vi "SI8.vi"(4 "error in":T13, 7 "Command":T14) -> (0 "error out":T13, 3 "Response":T11)   [LabVIEW 2018]
uses:
  MOKO_LabViewLibrary/MokoLowLevel/MokoLowLovelControl/MLLC_Command.ctl
  MOKO_LabViewLibrary/MokoLowLevel/MokoLowLovelControl/MLLC_Error.ctl
  MOKO_LabViewLibrary/MokoLowLevel/MokoLowLovelControl/MLLC_Mode.ctl
  MOKO_LabViewLibrary/MokoLowLevel/MokoLowLovelControl/MLLC_Response.ctl
  MOKO_LabViewLibrary/MokoLowLevel/MokoLowLovelControl/MLLC_DriverName.ctl
  MOKO_LabViewLibrary/MokoLowLevel/MokoLowLovelControl/MLLC_ResponseInit.ctl
  MOKO_LabViewLibrary/MokoLowLevel/MokoLowLovelControl/MLLC_Request.ctl
  MOKO_LabViewLibrary/MokoLowLevel/MokoLowLovelControl/MLLC_ErrorCode.ctl
  MOKO_LabViewLibrary/MokoLowLevel/MokoLowLovelControl/MLLC_ConnectCluster.ctl
  MOKO_LabViewLibrary/MokoLowLevel/MokoLowLovelControl/MLLC_InterfaceType.ctl
  MOKO_LabViewLibrary/MokoLowLevel/MokoLowLovelControl/MLLC_OpenedSession.ctl
  MOKO_LabViewLibrary/MokoLowLevel/MokoLowLovelControl/MLLC_InterfaceSettings.ctl
  MOKO_LabViewLibrary/MokoLowLevel/MokoLowLovelControl/MLLC_InterfaceKind.ctl
  MOKO_LabViewLibrary/MokoLowLevel/MokoLowLovelControl/MLLC_Rs232Settings.ctl
panel:
  in  "Settings":T6={"Permanent data"={"Connect"={"InterfaceType"=enum."VISA", "OpenedSession"="COM4", "InterfaceSettings"={"Interface"=enum."RS232", "EOS 4 read"=enum."Default (=EOS 4 write)", "EOS 4 write"=enum."CR (\\r)", "TMO, ms"=2000, "Sett"=variant(cluster{"Baud Rate":u32, "Data Bits":u16, "Parity":u16, "Stop Bits":u16, "Flow Control":u16, "Eho":bool} {"Baud Rate"=75, "Data Bits"=0, "Parity"=0, "Stop Bits"=0, "Flow Control"=0, "Eho"=FALSE})}}}, "Saved Data"=variant}
  in  "Error Code":T7=5420
  in  "Request":T8="?MOD"
  in  "ResponseInit":T9="XP2I"
  in  "Driver Name":T10="Crystal XP2"
  in  "Mode":T12=enum."Check"
  # "SI8"
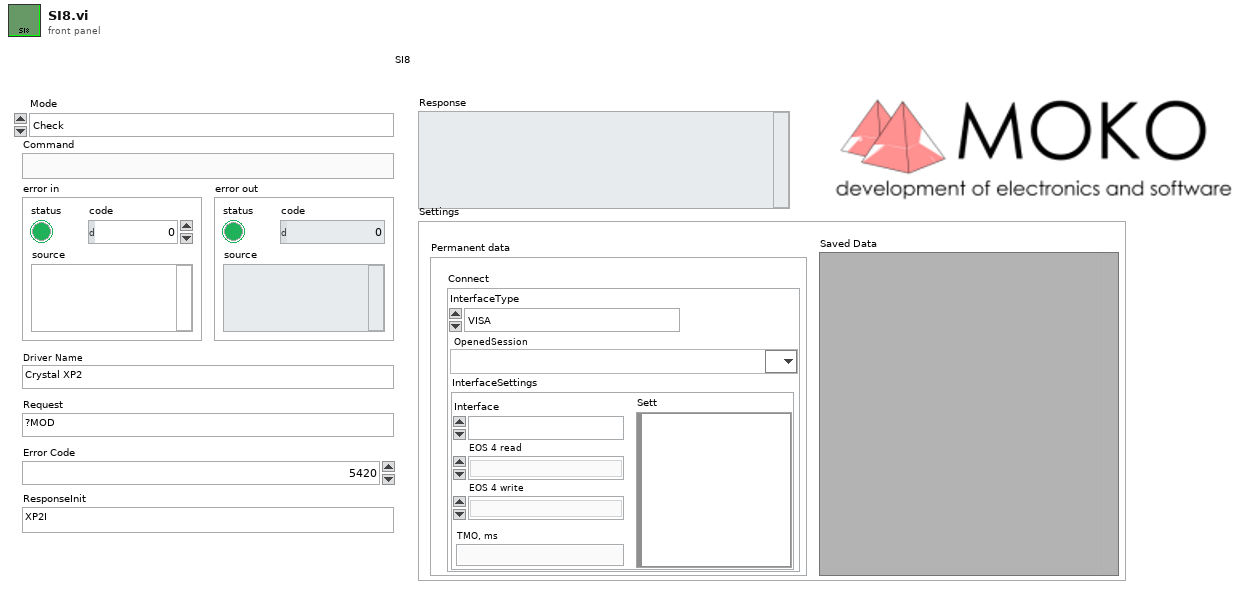
[diagram p1: front panel]
types:
  T1 = typedef "MLLC_ConnectCluster.ctl" = cluster{"InterfaceType":T2, "OpenedSession":T3, "InterfaceSettings":T4}
  T2 = typedef "MLLC_InterfaceType.ctl" = enum16{"VISA", "Prologix USB-GPIB"}
  T3 = typedef "MLLC_OpenedSession.ctl" = refnum<visa-resource-name>
  T4 = typedef "MLLC_InterfaceSettings.ctl" = cluster{"Interface":T5, "EOS 4 read":enum16{"Default (=EOS 4 write)", "CR (\\r)", "LF (\\n)", "None"}, "EOS 4 write":enum16{"CR+LF (\\r\\n)", "CR (\\r)", "LF (\\n)", "None"}, "TMO, ms":i32, "Sett":variant}
  T5 = typedef "MLLC_InterfaceKind.ctl" = enum16{"RS232", "GPIB", "USB", "Ethernet", "another"}
  T6 = cluster{"Permanent data":cluster{"Connect":T1}, "Saved Data":variant}
  T7 = typedef "MLLC_ErrorCode.ctl" = u32
  T8 = typedef "MLLC_Request.ctl" = string
  T9 = typedef "MLLC_ResponseInit.ctl" = string
  T10 = typedef "MLLC_DriverName.ctl" = string
  T11 = typedef "MLLC_Response.ctl" = string
  T12 = typedef "MLLC_Mode.ctl" = enum16{"get", "set", "close", "Init", "Check"}
  T13 = typedef "MLLC_Error.ctl" = errorcluster
  T14 = typedef "MLLC_Command.ctl" = string
  T15 = typedef "MLLC_Rs232Settings.ctl" = cluster{"Baud Rate":u32, "Data Bits":u16, "Parity":u16, "Stop Bits":u16, "Flow Control":u16, "Eho":bool, "Address":dbl}
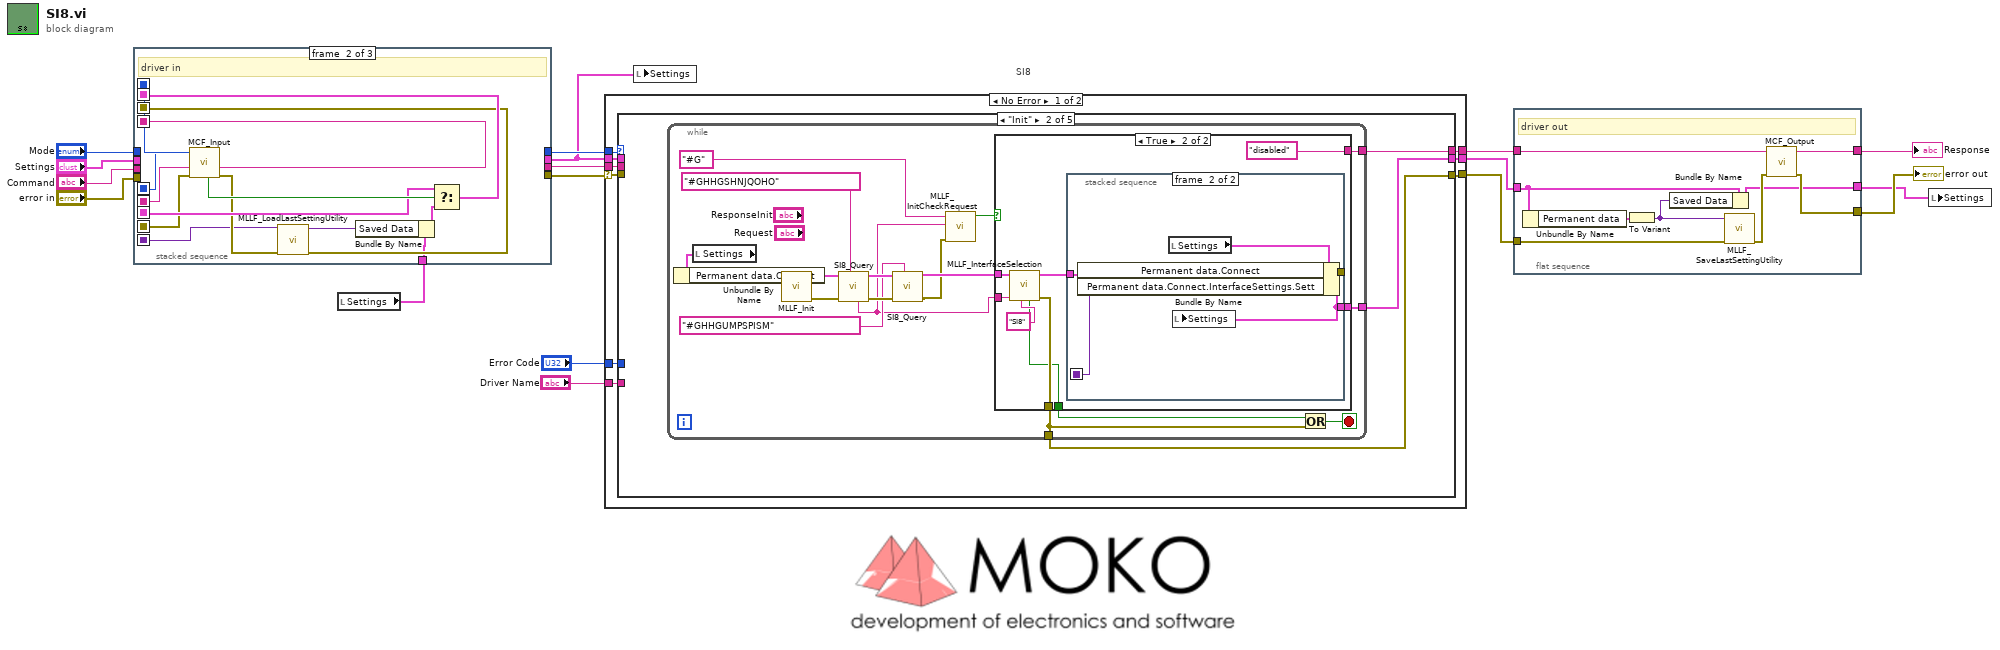
[diagram p0: block diagram]
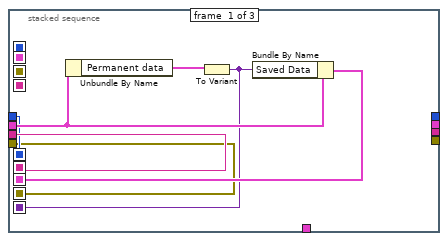
[diagram p2: hidden frame]
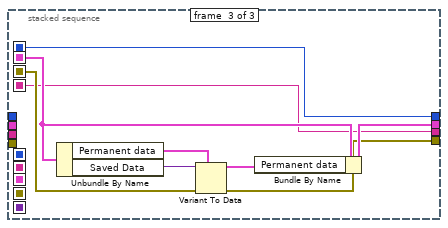
[diagram p3: hidden frame]
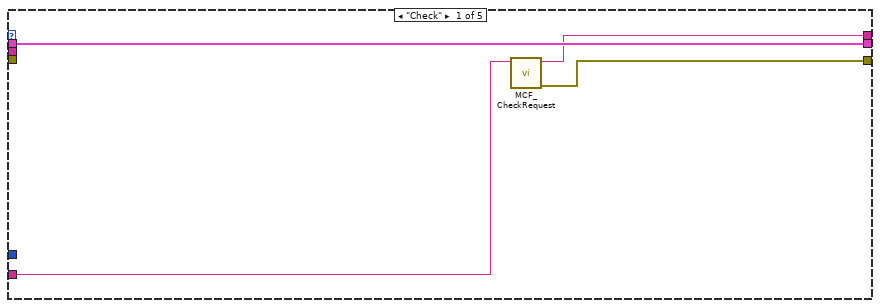
[diagram p4: hidden frame]
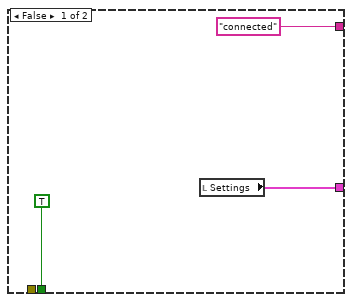
[diagram p5: hidden frame]
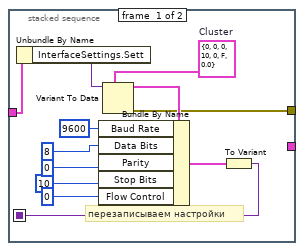
[diagram p6: hidden frame]
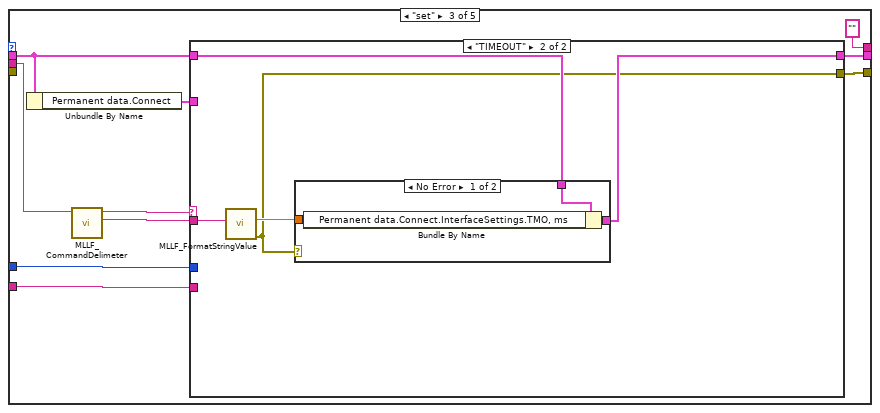
[diagram p7: hidden frame]
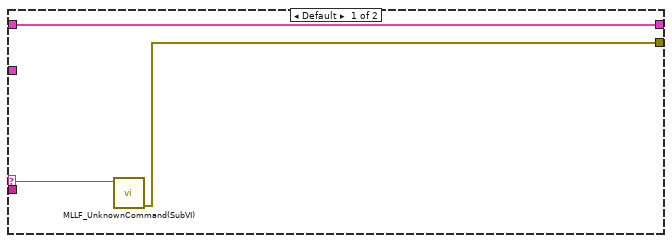
[diagram p8: hidden frame]
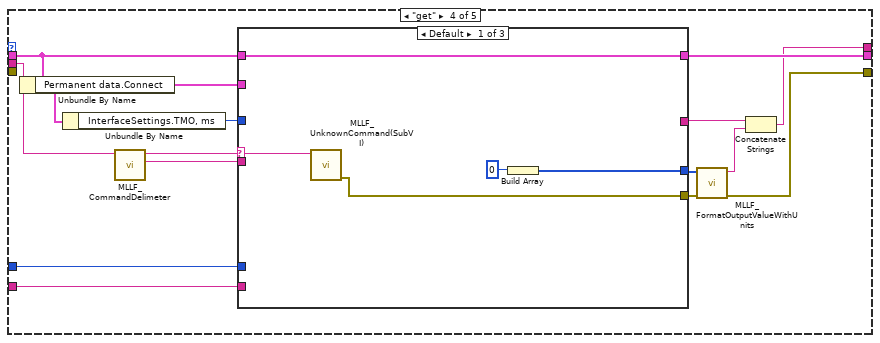
[diagram p10: hidden frame]
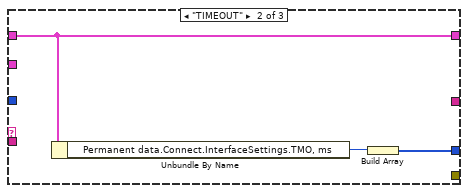
[diagram p11: hidden frame]
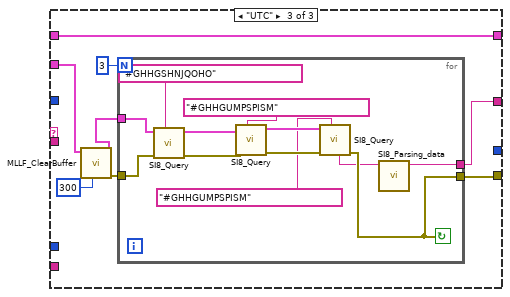
[diagram p12: hidden frame]
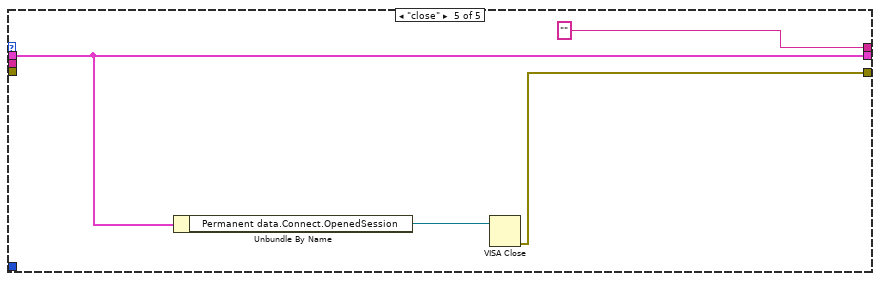
[diagram p13: hidden frame]
diagram:
  # "SI8"
  n1 = local read "Settings"() -> (w7:T6)
  n2 = stacked-sequence {
    seq-local: [w20 _ _] -> [_ w36 _]
    seq-local: [w19 _ _] -> [_ w37 _]
    seq-local: [w22 _ _] -> [_ w32 _]
    seq-local: [w18 _ _] -> [_ w31 _]
    seq-local: [w21 _ _] -> [_ w27 _]
    seq-local: [_ w28 _] -> [_ _ w44]
    seq-local: [_ w38 _] -> [_ _ w41]
    seq-local: [_ w35 _] -> [_ _ w40]
    seq-local: [_ w34 _] -> [_ _ w45]
    tunnel: "Command" -> [w20 _ _]
    tunnel: "Mode" -> [w19 _ _]
    tunnel: "error in" -> [w18 _ _]
    tunnel: "Settings" -> [w23 _ _]
    tunnel: w7 -> [_ w26 _]
    tunnel: [_ _ w40] -> w9
    tunnel: [_ _ w43] -> w10
    tunnel: [_ _ w42] -> w8
    tunnel: [_ _ w41] -> w11
    frame #0 {
      n3 = Unbundle By Name(w23) -> ("Permanent data"=w24:cluster{"Connect":T1})
      n4 = To Variant(anything=w24) -> (Variant=w21:variant)
      n5 = Bundle By Name(cluster=w23, "Saved Data"=w21) -> (w22:T6)
    }
    frame #1 {
      # "driver in"
      n6 = call "MCF_Input.vi"("Error In"=w31, "Command in"=w36, "Mode in"=w37) -> ("Error Out"=w30:errorcluster, "Command out"=w35:string, "Mode out"=w38:T12, "Boolean"=w33:bool)  [unwired: 5 in]
      n7 = call "MLLF_LoadLastSettingUtility.vi"("Error In"=w30, "Save data in"=w27) -> ("Error Out"=w28:errorcluster, "Save data out"=w25:variant)  [unwired: 8 in]
      n8 = Bundle By Name(cluster=w26, "Saved Data"=w25) -> (w29:T6)
      n9 = Select(t=w32, s=w33, f=w29) -> (s? t:f=w34:T6)
    }
    frame #2 {
      n10 = Unbundle By Name(w45) -> ("Permanent data"=w46:cluster{"Connect":T1}, "Saved Data"=w39:variant)
      n11 = Variant To Data(error in=w44, type=w46, Variant=w39) -> (data=w47:cluster{"Connect":T1}, error out=w42:errorcluster)
      n12 = Bundle By Name(cluster=w45, "Permanent data"=w47) -> (w43:T6)
    }
  }
  n13 = case shown="No Error" w8 {
    selector: w8 -> [w53 w179]
    tunnel: [w48 w179] -> w4
    tunnel: w11 -> [w56 _]
    tunnel: [w55 _] -> w6
    tunnel: w9 -> [w54 _]
    tunnel: w10 -> [w50 w178]
    tunnel: "Error Code" -> [w52 _]
    tunnel: "Driver Name" -> [w51 _]
    tunnel: [w49 w178] -> w5
    frame No Error {
      n14 = case shown="\"Init\"" w56 {
        tunnel: [w58 w63 "" ("Output String") w132 "" ("Output String")] -> w55
        tunnel: w54 -> [_ _ w112 w136 _]
        tunnel: w53 -> [_ _ _ _ _]
        tunnel: w52 -> [_ _ w118 w144 _]
        tunnel: w51 -> [w59 _ w115 w143 _]
        tunnel: w50 -> [w60 _ w117 w145 w176]
        tunnel: [w60 w62 w116 w142 w176] -> w49
        tunnel: [w57 w61 w109 w131 w175] -> w48
        frame "Check" {
          n15 = call "MCF_CheckRequest.vi"("Driver Name"=w59) -> ("Error Out"=w57:errorcluster, "Output String"=w58:string)  [unwired: 9 in]
        }
        frame "Init" {
          n16 = while {
            tunnel: [w78] -> w61
            tunnel: [w77] -> w63
            tunnel: [w76] -> w62
            stop <- w80 stop-if-true
            n17 = local read "Settings"() -> (w74:T6)
            n18 = Unbundle By Name(w74) -> ("Permanent data.Connect"=w73:T1)
            n19 = call "MLLF_Init.vi"("DriverConnect in"=w73) -> ("Error Out"=w81:errorcluster, "DriverConnect out"=w71:T1)  [unwired: 7 in]
            n20 = call "SI8_Query.vi"("String"="#GHHGSHNJQOHO", "error in (no error)"=w81, "DriverConnect in"=w71) -> ("error out"=w69:errorcluster, "DriverConnect out"=w68:T1, "String from device out"=w64:string)  [unwired: 6 in]
            n21 = call "SI8_Query.vi"("String"="#GHHGUMPSPISM", "error in (no error)"=w69, "DriverConnect in"=w68) -> ("error out"=w65:errorcluster, "DriverConnect out"=w66:T1)  [unwired: 6 in, 1 out]
            n22 = call "MLLF_InitCheckRequest.vi"("error in (no error)"=w65, "Answer"=w64, "Response Init"="#G") -> ("Design"=w75:bool)  [unwired: 5 in, 3 out]
            n23 = case shown="True" w75 {
              tunnel: w66 -> [_ w91]
              tunnel: [TRUE w87] -> w79
              tunnel: [_ w92] -> w78
              tunnel: ["connected" "disabled"] -> w77
              tunnel: [w82 w86] -> w76
              tunnel: w64 -> [_ w85]
              frame False {
                n24 = local read "Settings"() -> (w82:T6)
              }
              frame True {
                n25 = call "MLLF_InterfaceSelection.vi"("Driver Name"="SI8" ("String"), "Answer:"=w85, "DriverConnect in"=w91) -> ("error out"=w92:T13, "DriverConnect out"=w90:T1, "stop init?"=w87:bool)  [unwired: 4 in, 2 out]
                n26 = stacked-sequence {
                  seq-local: [w96 _] -> [_ w105]
                  tunnel: w90 -> [w94 w106]
                  tunnel: [w97 _] -> _
                  tunnel: [_ w107] -> w86
                  frame #0 {
                    w98 = T15 {"Baud Rate"=0, "Data Bits"=0, "Parity"=0, "Stop Bits"=10, "Flow Control"=0, "Eho"=FALSE, "Address"=0.0}  # Cluster
                    # "перезаписываем настройки"
                    n27 = Unbundle By Name(w94) -> ("InterfaceSettings.Sett"=w93:variant)
                    n28 = Variant To Data(type=w98, Variant=w93) -> (data=w99:T15, error out=w97:errorcluster)  [unwired: 1 in]
                    n29 = Bundle By Name(cluster=w99, "Baud Rate"=u32 9600, "Data Bits"=u16 8 ("Serial Settings:Data Bits"), "Parity"=u16 0 ("Serial Settings:Parity"), "Stop Bits"=u16 10 ("Serial Settings:Stop Bits"), "Flow Control"=u16 0 ("Serial Settings:Flow Control")) -> (w104:T15)
                    n30 = To Variant(anything=w104) -> (Variant=w96:variant)
                  }
                  frame #1 {
                    n31 = local read "Settings"() -> (w108:T6)
                    n32 = Bundle By Name(cluster=w108, "Permanent data.Connect"=w106, "Permanent data.Connect.InterfaceSettings.Sett"=w105) -> (w107:T6)
                    n33 = local write "Settings"(w107) -> ()
                  }
                }
              }
            }
            n34 = Or(x=w79, y=w78) -> (x .or. y?=w80:bool)
          }
        }
        frame "set" {
          n35 = Unbundle By Name(w117) -> ("Permanent data.Connect"=w113:T1)
          n36 = call "MLLF_CommandDelimeter.vi"("command with param"=w112) -> ("param 1"=w110:string, "command"=w111:string)  [unwired: 6 in, 3 out]
          n37 = case shown="\"TIMEOUT\"" w111 {
            selector: w111 -> [w120 _]
            tunnel: w110 -> [_ w124]
            tunnel: w118 -> [_ _]
            tunnel: w117 -> [w121 w125]
            tunnel: [w121 w126] -> w116
            tunnel: w115 -> [_ _]
            tunnel: [w119 w122] -> w109
            tunnel: w113 -> [_ _]
            frame Default {
              n38 = call "MLLF_UnknownCommand(SubVI).vi"("Unknown command"=w120) -> ("error out"=w119:errorcluster)  [unwired: 10 in]
            }
            frame "TIMEOUT" {
              n39 = call "MLLF_FormatStringValue.vi"("String Value"=w124) -> ("error out"=w122:T13, "number"=w123:dbl)  [unwired: 8 in, 1 out]
              n40 = case shown="No Error" w122 {
                tunnel: [w129 w130] -> w126
                tunnel: w125 -> [w128 w130]
                tunnel: w123 -> [w127 _]
                frame No Error {
                  n41 = Bundle By Name(cluster=w128, "Permanent data.Connect.InterfaceSettings.TMO, ms"=w127) -> (w129:T6)
                }
                frame Error {
                }
              }
            }
          }
        }
        frame "get" {
          n42 = Unbundle By Name(w145) -> ("Permanent data.Connect"=w135:T1)
          n43 = Unbundle By Name(w135) -> ("InterfaceSettings.TMO, ms"=w139:i32)
          n44 = call "MLLF_CommandDelimeter.vi"("command with param"=w136) -> ("param 1"=w133:string, "command"=w134:string)  [unwired: 6 in, 3 out]
          n45 = case shown="Default" w134 {
            selector: w134 -> [w147 _ _]
            tunnel: w133 -> [_ _ _]
            tunnel: [w146 _ w158] -> w141
            tunnel: w144 -> [_ _ _]
            tunnel: [w150 w153 w161] -> w142
            tunnel: w145 -> [w150 w153 w161]
            tunnel: [w148 w151 _] -> w140
            tunnel: w143 -> [_ _ _]
            tunnel: w139 -> [_ _ _]
            tunnel: [_ _ w160] -> w137
            tunnel: w135 -> [_ _ w157]
            frame Default {
              n46 = call "MLLF_UnknownCommand(SubVI).vi"("Unknown command"=w147) -> ("error out"=w146:errorcluster)  [unwired: 10 in]
              n47 = Build Array(0 ("TimeOut")) -> (w148:i32[])
            }
            frame "TIMEOUT" {
              n48 = Unbundle By Name(w153) -> ("Permanent data.Connect.InterfaceSettings.TMO, ms"=w152:i32)
              n49 = Build Array(w152) -> (w151:i32[])
            }
            frame "UTC" {
              n50 = call "MLLF_ClearBuffer.vi"("Timeout(default = 300 ms)"=u32 300 ("Timeout"), "DriverConnect in"=w157) -> ("Error Out"=w154:errorcluster, "DriverConnect out"=w155:T1)  [unwired: 6 in, 1 out]
              n51 = for {
                N: 3 -> [_]
                tunnel: w155 -> [w173]
                tunnel: [w163] -> w160
                tunnel: [w165] -> w158
                tunnel: w154 -> [w162]
                stop <- w165 continue-if-true
                n52 = call "SI8_Query.vi"("String"="#GHHGSHNJQOHO", "error in (no error)"=w162, "DriverConnect in"=w173) -> ("error out"=w171:errorcluster, "DriverConnect out"=w170:T1)  [unwired: 6 in, 1 out]
                n53 = call "SI8_Query.vi"("String"="#GHHGUMPSPISM", "error in (no error)"=w171, "DriverConnect in"=w170) -> ("error out"=w169:errorcluster, "DriverConnect out"=w168:T1)  [unwired: 6 in, 1 out]
                n54 = call "SI8_Query.vi"("String"="#GHHGUMPSPISM", "error in (no error)"=w169, "DriverConnect in"=w168) -> ("error out"=w165:errorcluster, "String from device out"=w164:string)  [unwired: 6 in, 1 out]
                n55 = call "SI8_Parsing_data.vi"("IN"=w164) -> ("OUT"=w163:string)  [unwired: 10 in]
              }
            }
          }
          n56 = call "MLLF_FormatOutputValueWithUnits.vi"("error in"=w141, "ValuesIn"=w140) -> ("error out"=w131:T13, "Result string"=w138:T14)  [unwired: 8 in]
          n57 = Concatenate Strings(w137, w138) -> (w132:string)
        }
        frame "close" {
          n58 = Unbundle By Name(w176) -> ("Permanent data.Connect.OpenedSession"=w177:T3)
          n59 = VISA Close(VISA resource name=w177) -> (error out=w175:errorcluster)  [unwired: 1 in]
        }
      }
    }
    frame Error {
    }
  }
  n60 = local write "Settings"(w10) -> ()
  n61 = flat-sequence {
    tunnel: [w188] -> w3
    tunnel: [w187] -> w2
    tunnel: w6 -> [w186]
    tunnel: w4 -> [w185]
    tunnel: w5 -> [w181]
    tunnel: [w183] -> w1
    frame #0 {
      # "driver out"
      n62 = Unbundle By Name(w181) -> ("Permanent data"=w180:cluster{"Connect":T1})
      n63 = To Variant(anything=w180) -> (Variant=w182:variant)
      n64 = Bundle By Name(cluster=w181, "Saved Data"=w182) -> (w183:T6)
      n65 = call "MLLF_SaveLastSettingUtility.vi"("error in"=w185, "Saved Data"=w182) -> ("error out"=w184:T13)  [unwired: 8 in, 1 out]
      n66 = call "MCF_Output.vi"("Error In"=w184, "Input"=w186) -> ("Error Out"=w187:errorcluster, "Output"=w188:string)  [unwired: 8 in]
    }
  }
  n67 = local write "Settings"(w1) -> ()
  "error out" <- w2
  "Response" <- w3
